vi "Test Call Assertion Type Recorded on Failing Pass If Equal.vi"(8 "error in (no error)":errorcluster, 11 "Test Case In":refnum<class "Test Case V2 Assertions Test.lvclass">) -> (0 "error out":errorcluster, 3 "Test Case Out":refnum<class "Test Case V2 Assertions Test.lvclass">)   [LabVIEW 2020, in "Test Case V2 Assertions Test.lvclass"]
uses:
  Test Case V2 Assertions Test.lvclass
  C:/Program Files (x86)/National Instruments/LabVIEW 2020/vi.lib/Astemes/LUnit/Test Case.lvclass
  Result/Type.ctl
  LUnit Test Case Tests/LUnit Test Case V2 Test Double/Methods.ctl
  <vilib>/Astemes/LUnit/Test Case.lvclass/Test Case.ctl
  e8c5eeff-a694-4c0d-b261-74e2e6f5327d.vi
  <vilib>/Astemes/LUnit/Palette/Pass.vi
  <vilib>/Astemes/LUnit/Palette/Fail.vi
  <vilib>/Astemes/LUnit/Compare Variants.vi
  <vilib>/Astemes/LUnit/Describe Comparison.vi
  <vilib>/Astemes/LUnit/Set Assertion Type.vi
  <vilib>/Astemes/LUnit/Add test result.vi
  <vilib>/Astemes/LUnit/Variant to string.vi
  <vilib>/Astemes/LUnit/LUnit Record Assertion Result.vi
  <vilib>/Astemes/LUnit/LUnit Aggregate Assertion Results.vi
  <vilib>/Astemes/LUnit/Method Result/LUnit Merge Status.vi
  <vilib>/Astemes/LUnit/LUnit Concatenate result strings.vi
  <vilib>/Utility/Data Type/Get Type Information.vi
  <vilib>/Utility/LVClass/Get LV Class Name.vi
  LUnit Test Case/LUnit Test Case V2.lvclass
  LUnit Test Case Tests/LUnit Test Case V2 Test Double/LUnit Test Case V2 Test Double.lvclass
  Result/Result.lvlib
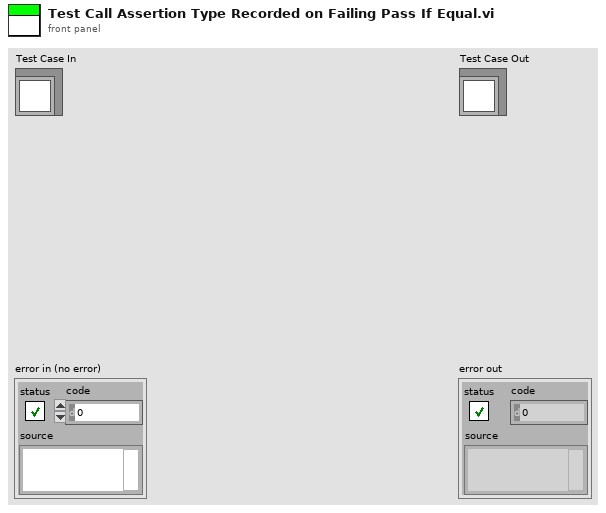
[diagram p1: front panel]
types:
  T1 = typedef "LUnit Test Case V2 Test Double.lvclass/Methods.ctl" = enum16{"Test Failing Test.vi", "Test Passing Test.vi", "Test Error Test.vi", "Test Skip Test.vi", "Test Passing Pass If Test.vi", "Test Failing Pass If Test.vi", "Test Failing Fail If Test.vi", "Test Passing Fail If Test.vi", "Test Passing Pass If Error Test.vi", "Test Failing Pass If Error Test.vi", "Test Passing Fail If Error Test.vi", "Test Failing Fail If Error Test.vi", "Test Passing Pass If Equal Test.vi", "Test Failing Pass If Equal Test.vi", "Test Failing Fail If Equal Test.vi", "Test Passing Fail If Equal Test.vi"}
  T2 = typedef "Result.lvlib/Type.ctl" = enum16{"Method", "Case", "Suite", "Pass", "Fail", "Skip", "Pass if", "Fail if", "Pass if Error", "Fail if Error", "Pass if Equal", "Fail if Equal"}
  T3 = typedef "Result.lvlib/Result.ctl" = cluster{"Case":string, "Message":string, "Description":string, "Status":T4, "Result Type":T2, "Execution Time":dbl}
  T4 = typedef "Result.lvlib/Status.ctl" = enum16{"Passed", "Failed", "Error", "Skipped", "Setup Error", "Broken", "Teardown Error"}
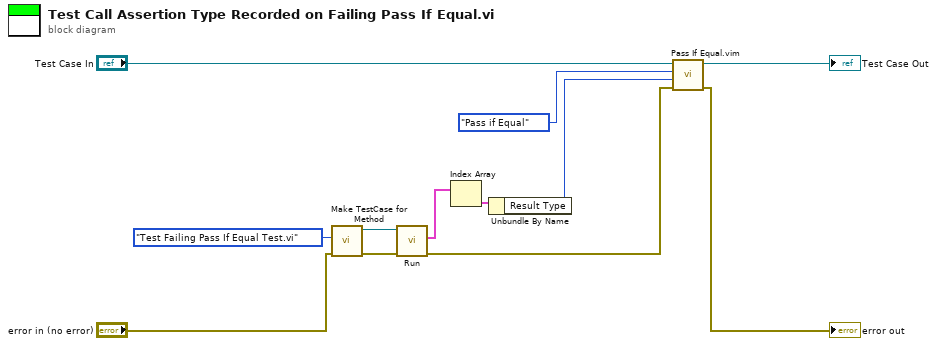
[diagram p0: block diagram]
diagram:
  n1 = call "Make TestCase for Method.vi"("error in (no error)"="error in (no error)", "Test Method"=Methods."Test Failing Pass If Equal Test.vi") -> ("error out"=w8:errorcluster, "LUnit Test Case V2 out"=w9:refnum<class "LUnit Test Case V2.lvclass">)  [unwired: 8 in]
  n2 = call-dynamic "Run.vi"("error in (no error)"=w8, "LUnit Test Case V2 in"=w9) -> ("error out"=w6:errorcluster, "Results"=w5:T3[])  [unwired: 8 in]
  n3 = Index Array(array=w5) -> (element=w4:T3)  [unwired: 1 in]
  n4 = Unbundle By Name(w4) -> ("Result Type"=w3:T2)
  n5 = call "Pass If Equal.vim"("error in (no error)"=w6, "Actual"=w3, "Expected"=Type."Pass if Equal" ("Result Type"), "LUnit Test Case In"="Test Case In") -> ("error out"=→"error out":errorcluster, "LUnit Test Case Out"=→"Test Case Out":refnum<class "Test Case V2 Assertions Test.lvclass">)  [unwired: 6 in]
